vi "transform MessageMeasurement.vi"(11 "measurements (KVP)":variant) -> (3 "measurements (Attributes)":variant)   [LabVIEW 2020, in "Caraya.lvlib" / "Test Event Storage.lvclass"]
uses:
  Test Event Storage.lvclass
  Test Manager Message Measurement/TestManagerMsg.Measurement.lvclass
  Test Manager Message Measurement/TestManagerMsg.Measurement.lvclass/TestManagerMsg.Measurement.ctl
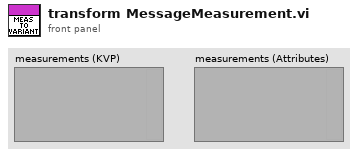
[diagram p1: front panel]
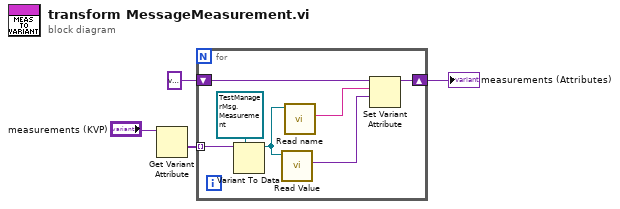
[diagram p0: block diagram]
diagram:
  n1 = Get Variant Attribute(Variant="measurements (KVP)") -> (values=w2:variant[])  [unwired: 3 in, 3 out]
  n2 = for {
    tunnel: w2 -> [w11] mode=indexing
    shift-right: [w10] -> w4
    shift-left: variant ("properties") -> [w9]
    n3 = Variant To Data(type=refnum<class "TestManagerMsg.Measurement.lvclass"> refnum ("Caraya.lvlib:TestManagerMsg.Measurement.lvclass"), Variant=w11) -> (data=w7:refnum<class "TestManagerMsg.Measurement.lvclass">)  [unwired: 1 in, 1 out]
    n4 = call "Read Value.vi"("TestManagerMsg.Measurement in"=w7) -> ("Value"=w5:variant)  [unwired: 9 in, 1 out]
    n5 = call "Read name.vi"("TestManagerMsg.Measurement in"=w7) -> ("name"=w6:string)  [unwired: 9 in, 1 out]
    n6 = Set Variant Attribute(Variant=w9, name=w6, value=w5) -> (Variant out=w10:variant)  [unwired: 1 in, 2 out]
  }
  "measurements (Attributes)" <- w4
